vi "set_start_daq_flag.vi"(8 "error in (no error)":errorcluster, 10 "start daq from within imagingMode?":bool, 11 "ImagingModeDL090923Scaffold in":refnum<class "ImagingModeDL090923Scaffold.lvclass">) -> (0 "error out":errorcluster, 3 "ImagingModeDL090923Scaffold out":refnum<class "ImagingModeDL090923Scaffold.lvclass">)   [LabVIEW 2010, in "ImagingModeDL090923Scaffold.lvclass"]
uses:
  ImagingModeDL090923Scaffold.lvclass
  ImagingModeDL090923Scaffold.lvclass/ImagingModeDL090923Scaffold.ctl
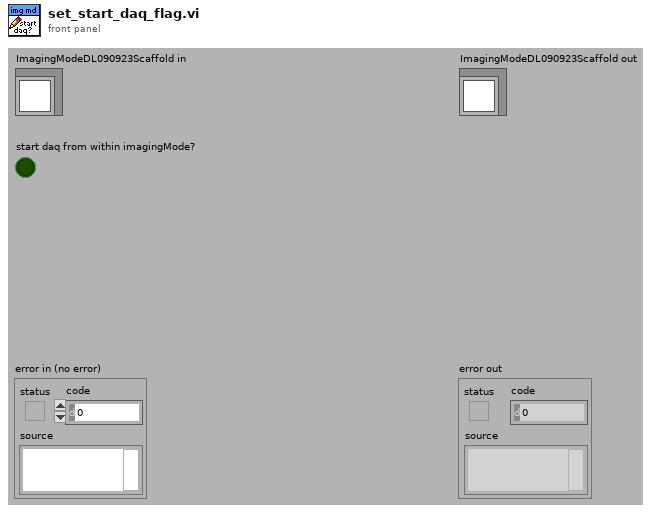
[diagram p1: front panel]
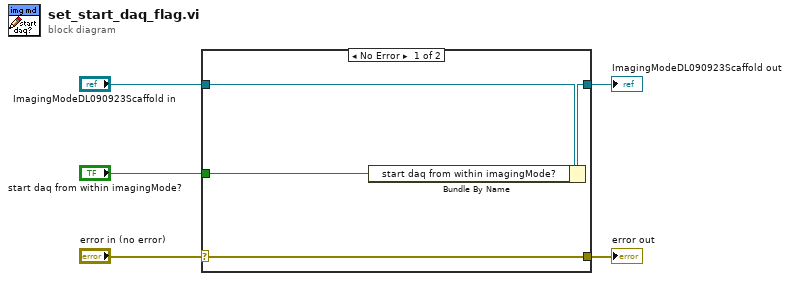
[diagram p0: block diagram]
diagram:
  n1 = case shown="No Error" "error in (no error)" {
    selector: "error in (no error)" -> [w9 w10]
    tunnel: [w9 w10] -> w4
    tunnel: [w7 w11] -> w2
    tunnel: "ImagingModeDL090923Scaffold in" -> [w8 w11]
    tunnel: "start daq from within imagingMode?" -> [w6 _]
    frame No Error {
      n2 = Bundle By Name(cluster=w8, "start daq from within imagingMode?"=w6) -> (w7:refnum<class "ImagingModeDL090923Scaffold.lvclass">)
    }
    frame Error {
    }
  }
  "error out" <- w4
  "ImagingModeDL090923Scaffold out" <- w2
